vi "FindTag.vi"(8 "error in (no error)":errorcluster, 10 "Tag":string, 11 "ToolStripItem":refnum<k24>) -> (0 "error out":errorcluster, 2 "Found":bool, 3 "ToolStripItem out":refnum<k24>)   [LabVIEW 2019, in "MGI_ToolStrip.lvclass"]
uses:
  MGI_ToolStrip.lvclass
  System.Windows.Forms
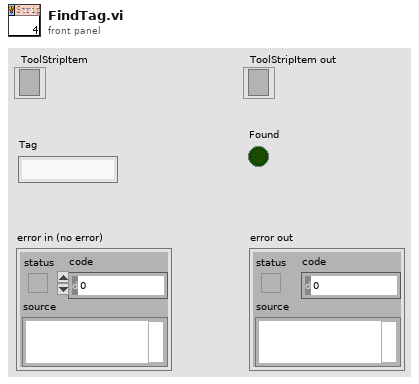
[diagram p1: front panel]
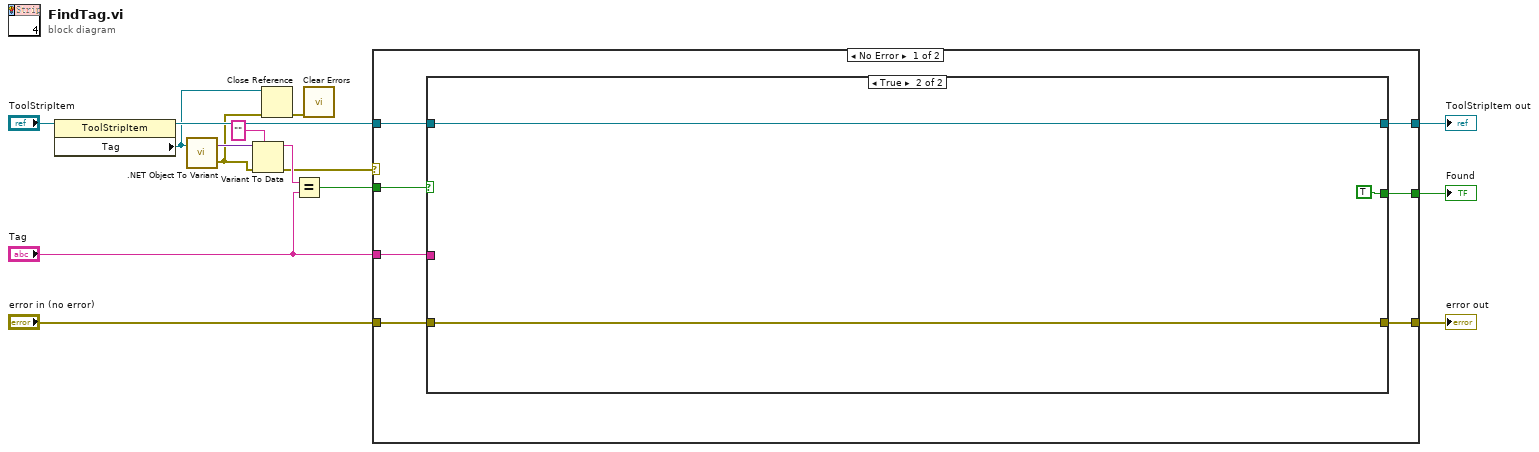
[diagram p0: block diagram]
diagram:
  n1 = property class="ToolStripItem"(reference="ToolStripItem") -> (reference out=w9:refnum<k24>, "Tag"=w4:refnum<k24>)  [unwired: 1 in, 1 out]
  n2 = call <vilib>:".NET Object To Variant.vi"(".NET object"=w4) -> ("error out"=w3:errorcluster, "variant"=w14:variant)  [unwired: 1 in]
  n3 = Variant To Data(error in=w3, type="", Variant=w14) -> (data=w12:string, error out=w1:errorcluster)
  n4 = Close Reference(reference=w4, error in (no error)=w3) -> (error out=w2:errorcluster)
  n5 = Equal?(x=w12, y="Tag") -> (x = y?=w11:bool)
  n6 = call <vilib>:"Clear Errors.vi"("error in (no error)"=w2) -> ()  [unwired: 5 in, 2 out]
  n7 = case shown="No Error" w1 {
    tunnel: w11 -> [w22 _]
    tunnel: [w21 _] -> w10
    tunnel: w9 -> [w20 _]
    tunnel: [w19 _] -> w8
    tunnel: [w18 w27] -> w7
    tunnel: "error in (no error)" -> [w17 w27]
    tunnel: "Tag" -> [w16 _]
    frame No Error {
      n8 = case shown="True" w22 {
        tunnel: [_ w26] -> w21
        tunnel: w20 -> [_ w26]
        tunnel: [_ TRUE] -> w19
        tunnel: [w23 w24] -> w18
        tunnel: w17 -> [w23 w24]
        tunnel: w16 -> [_ _]
        frame False {
        }
        frame True {
        }
      }
    }
    frame Error {
    }
  }
  "error out" <- w7
  "ToolStripItem out" <- w10
  "Found" <- w8
